vi "LC1_MS_Main_for_AEROS.vi"(0 "MS_Network_Settings":T12, 1 "Analog Output":T5(array[cluster]) {"analog info"."value" format="%#_15f"; "variation" items=["32-bit"=1, "16-bit"=2, "Single-prec"=3, "Double-prec"=4]; "mode" items=["SBO"=0, "Select"=3, "Operate"=4, "Direct"=5, "Direct No Ack"=6]}, 2 "Analog Input Index":cluster{"start":u16, "variation (Default)":T1}[](array[cluster]) {"variation (Default)" items=["Default", "32-bit with Flag", "16-bit with Flag", "32-bit without Flag", "16-bit without Flag", "Single-prec with Flag", "Double-prec with Flag"]}, 3 "Digital Input Indexes":u16[](array[numeric]), 5 "input cluster":T16={"Binary Out Mode"=6, "Binary In Variation"=0, "Analog Out Variation"=4, "Analog Out Mode"=6, "Analog In Variation"=6} {"Binary Out Mode" items=["SBO"=0, "Select"=3, "Operate"=4, "Direct"=5, "Direct No Ack"=6]; "Binary In Variation" items=["Default", "Packed Format", "With Flags"]; "Analog Out Variation" items=["32-bit"=1, "16-bit"=2, "Single-prec"=3, "Double-prec"=4]; "Analog Out Mode" items=["SBO"=0, "Select"=3, "Operate"=4, "Direct"=5, "Direct No Ack"=6]; "Analog In Variation" items=["Default", "32-bit with Flag", "16-bit with Flag", "32-bit without Flag", "16-bit without Flag", "Single-prec with Flag", "Double-prec with Flag"]}, 7 "MS_RESET":bool, 9 "MS_ENABLE":bool, 11 "Poll Enable":T13, 12 "DNP3 Session feedback":T15, 13 "Digital Output":T6[](array[typedef]) {"CROB value"."Control" items=["Nul"=0, "Pulse On"=1, "Pulse Off"=2, "Latch On"=3, "Latch Off"=4, "Close"=65, "Trip"=129]}) -> (4 "MS_SETTINGS_CHANGED":bool, 6 "MS_RESET_IND":bool, 8 "Cluster":T14, 10 "Analog Input":dbl[](array[numeric]), 14 "DNP3 Session":T15, 15 "Digital Input":bool[](array[boolean]))   [LabVIEW 2016]
uses:
  Tab_Master.ctl
  <vilib>/DNP3/DNP3_Master/Operation Mode.ctl
  <vilib>/DNP3/DNP3_Master/Poll Binary Input Variation.ctl
  <vilib>/DNP3/DNP3_Master/Analog Variation.ctl
  <vilib>/DNP3/DNP3_Master/Poll Analog Input Variation.ctl
  <vilib>/DNP3/DNP3_Master/Response Type.ctl
  <vilib>/DNP3/DNP3_Master/Start Stop.ctl
  <vilib>/DNP3/DNP3_Master/Crob With Index.ctl
  <vilib>/DNP3/DNP3_Common/crob.ctl
  <vilib>/DNP3/DNP3_Common/crob_ctrl.ctl
  <vilib>/DNP3/DNP3_Master/Analog Info.ctl
  <vilib>/Utility/error.llb/Error Cluster From Error Code.vi
  <vilib>/DNP3/DNP3_Master/Send Poll Analog Input By StartStop (Blocking).vi
  <vilib>/DNP3/DNP3_Master/Read Analog Input.vi
  <vilib>/DNP3/DNP3_Master/Send Analog Output Block (Blocking).vi
  <vilib>/DNP3/DNP3_Master/Send Poll Binary Input By StartStop (Blocking).vi
  <vilib>/DNP3/DNP3_Master/Read Binary Input.vi
  <vilib>/DNP3/DNP3_Master/Send CROB (Blocking).vi
  <vilib>/ErrorRing/Error Ring.xnode
  <vilib>/DNP3/DNP3_Master.lvlib
  <resource>/objmgr/dnp3.rc
  DNP3_Master_Station_MGCC.lvlib
  <vilib>/DNP3/DNP3_Common.lvlib
panel:
  out "PollD":T9[](array[typedef])
  out "Binary Out Mode":T4=6 items=["SBO"=0, "Select"=3, "Operate"=4, "Direct"=5, "Direct No Ack"=6]
  out "Binary In Variation":T10 items=["Default", "Packed Format", "With Flags"]
  out "Analog Out Variation":T3=4 items=["32-bit"=1, "16-bit"=2, "Single-prec"=3, "Double-prec"=4]
  out "Analog Out Mode":T4 items=["SBO"=0, "Select"=3, "Operate"=4, "Direct"=5, "Direct No Ack"=6]
  out "Analog In Variation":T1 items=["Default", "32-bit with Flag", "16-bit with Flag", "32-bit without Flag", "16-bit without Flag", "Single-prec with Flag", "Double-prec with Flag"]
  out "MS_TX_Status_Binary":T11
  out "MS_TX_Status_Analog":T11
  out "MS_RX_Status_Binary":T11
  out "MS_RX_Status_Analog":T11
  out "MS_Network_Settings_Initial":T12
  in  "En_Tx_Di":bool
  in  "En_Tx_An":bool
  in  "En_Rx_Di":bool
  in  "En_Rx_An":bool
  out "object flags":u8[](array[numeric]) format="%08b"
  in  "Channel Setting":T17
  in  "serial port":u16=1
  in  "baud rate (9600)":u32=9600
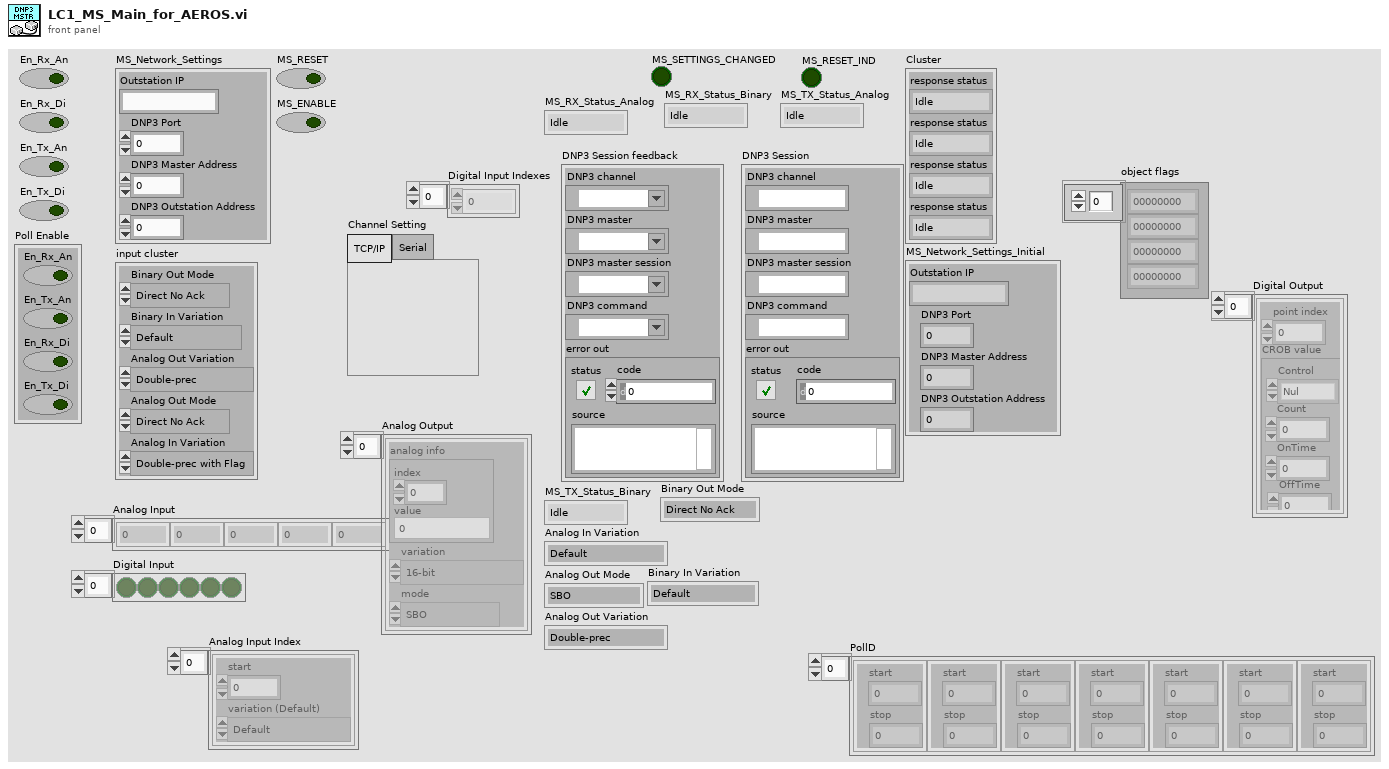
[diagram p1: front panel]
types:
  T1 = typedef "DNP3_Master.lvlib/Poll Analog Input Variation.ctl" = u8
  T2 = typedef "DNP3_Master.lvlib/Analog Info.ctl" = cluster{"index":u16, "value":dbl}
  T3 = typedef "DNP3_Master.lvlib/Analog Variation.ctl" = u8
  T4 = typedef "DNP3_Master.lvlib/Operation Mode.ctl" = u8
  T5 = cluster{"analog info":T2, "variation":T3, "mode":T4}[]
  T6 = typedef "DNP3_Master.lvlib/Crob With Index.ctl" = cluster{"point index":u16, "CROB value":T7}
  T7 = typedef "DNP3_Common.lvlib/crob.ctl" = cluster{"OnTime":u32, "Count":u8, "OffTime":u32, "Control":T8}
  T8 = typedef "DNP3_Common.lvlib/crob_ctrl.ctl" = u8
  T9 = typedef "DNP3_Master.lvlib/Start Stop.ctl" = cluster{"start":u16, "stop":u16}
  T10 = typedef "DNP3_Master.lvlib/Poll Binary Input Variation.ctl" = u8
  T11 = typedef "DNP3_Master.lvlib/Response Type.ctl" = enum16{"Idle", "Buffering", "Pending", "Success", "Failure", "Mismatch", "Status Code", "IIN", "Timeout", "Cancel"}
  T12 = cluster{"Outstation IP":string, "DNP3 Port":u16, "DNP3 Master Address":u16, "DNP3 Outstation Address":u16}
  T13 = cluster{"En_Rx_An":bool, "En_Tx_An":bool, "En_Rx_Di":bool, "En_Tx_Di":bool}
  T14 = cluster{"response status":T11, "response status":T11, "response status":T11, "response status":T11}
  T15 = cluster{"DNP3 channel":refnum<k21>, "DNP3 master":refnum<k21>, "DNP3 master session":refnum<k21>, "DNP3 command":refnum<k21>, "error out":errorcluster}
  T16 = cluster{"Binary Out Mode":T4, "Binary In Variation":T10, "Analog Out Variation":T3, "Analog Out Mode":T4, "Analog In Variation":T1}
  T17 = typedef "Tab_Master.ctl" = enum32{"TCP/IP", "Serial"}
  T18 = cluster{"Analog RX":T11, "Analog RX":T11, "Analog RX":T11, "Analog RX":T11}
  T19 = cluster{"DNP3 Master Address":u16, "DNP3 Outstation Address":u16}
  T20 = cluster{bool, "Outstation IP":string, "DNP3 Port":u16, "serial port":u16, "baud rate (9600)":u32}
  T21 = cluster{"MS_RX_Status_Analog":T11, "MS_TX_Status_Analog":T11, "MS_RX_Status_Binary":T11, "MS_TX_Status_Binary":T11}
  T22 = cluster{"DNP3 channel":refnum<k21>, "DNP3 master":refnum<k21>, "DNP3 master session":refnum<k21>, "DNP3 command":refnum<k21>, "error IO":errorcluster}
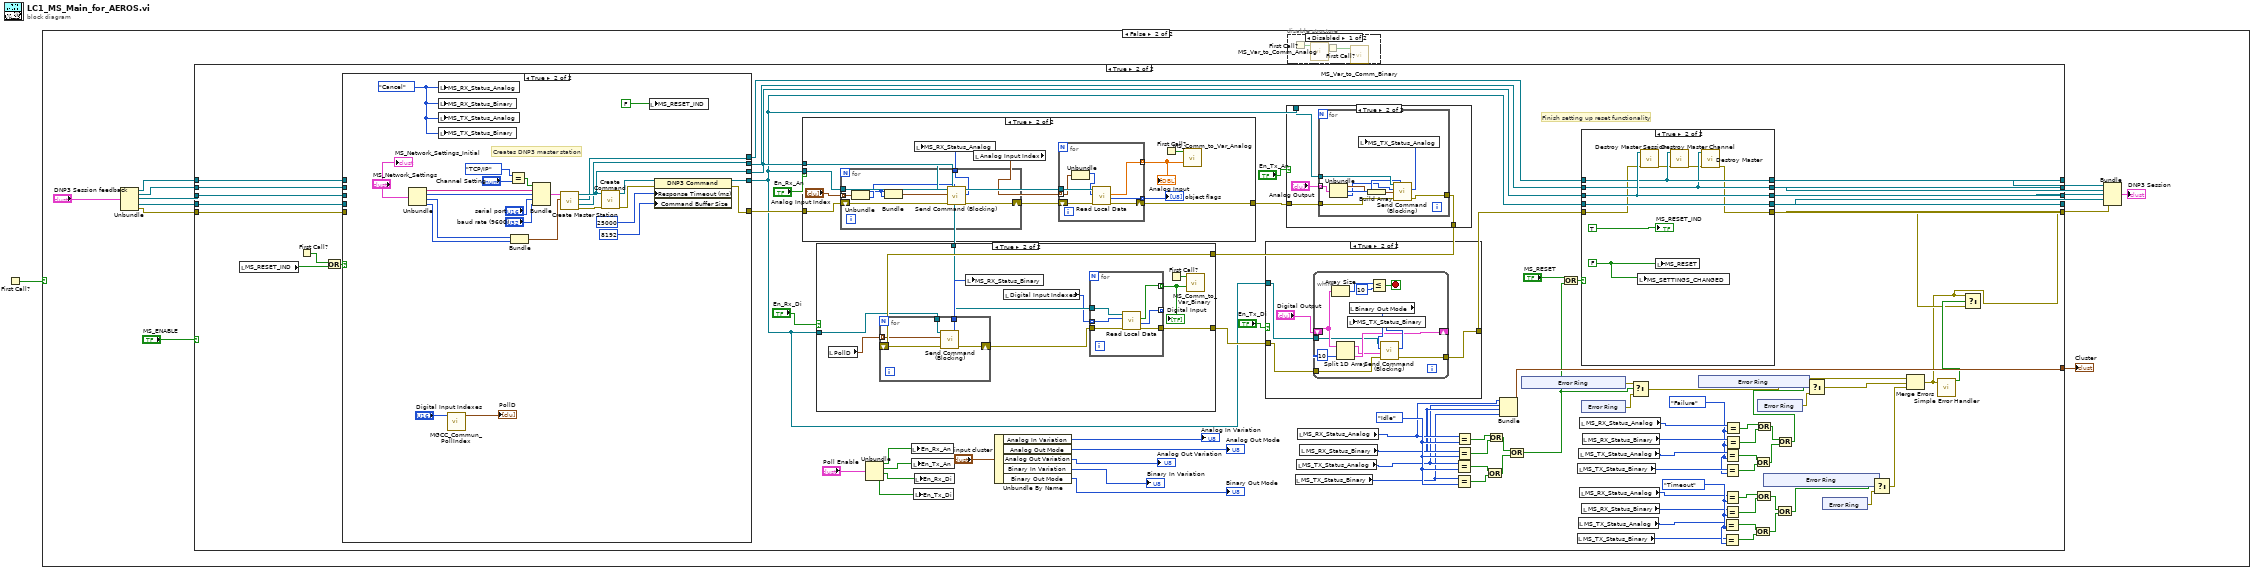
[diagram p0: block diagram]
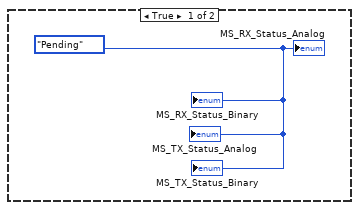
[diagram p2: hidden frame]
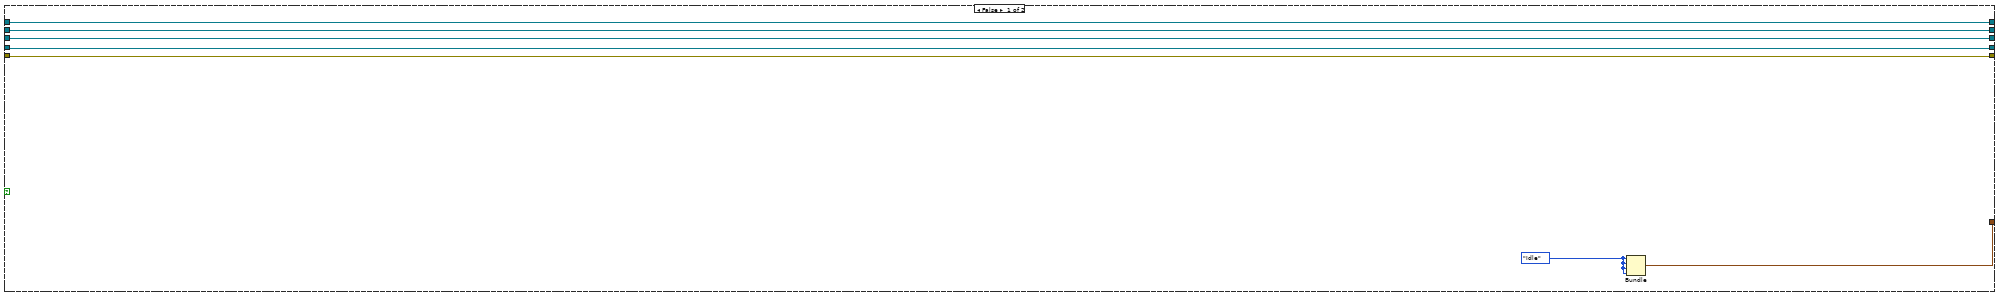
[diagram p4: hidden frame]
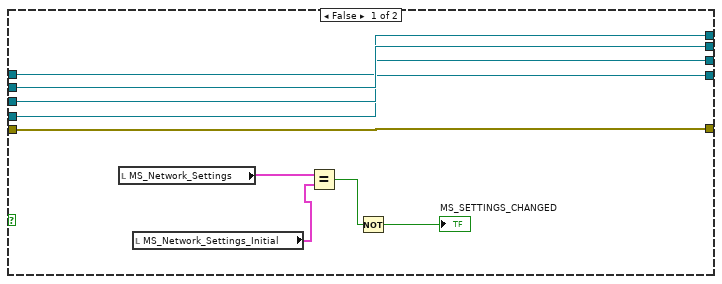
[diagram p10: hidden frame]
diagram:
  n1 = First Call?() -> (First Call?: T/F=w1:bool)
  n2 = case shown="False" w1 {
    frame True {
      w2 = Response_Type."Pending" ("LC1_MS_RX_Status_Binary")
      "MS_RX_Status_Analog" <- w2
      "MS_RX_Status_Binary" <- w2
      "MS_TX_Status_Analog" <- w2
      "MS_TX_Status_Binary" <- w2
    }
    frame False {
      n3 = Unbundle("DNP3 Session feedback") -> ("DNP3 channel"=w16:refnum<k21>, "DNP3 master"=w15:refnum<k21>, "DNP3 master session"=w13:refnum<k21>, "DNP3 command"=w14:refnum<k21>, "error out"=w12:errorcluster)
      n4 = case shown="True" "MS_ENABLE" {
        tunnel: w15 -> [w25 w109]
        tunnel: w13 -> [w24 w108]
        tunnel: w14 -> [w23 w107]
        tunnel: [w25 w105] -> w7
        tunnel: w12 -> [w22 w104]
        tunnel: [w22 w26] -> w4
        tunnel: [w24 w103] -> w6
        tunnel: [w23 w101] -> w5
        tunnel: [w21 w90] -> w8
        tunnel: w16 -> [w21 w89]
        tunnel: [w20 w85] -> w9
        frame False {
          w19 = Response_Type."Idle" ("Analog RX")
          n5 = Bundle("Analog RX"=w19, "Analog RX"=w19, "Analog RX"=w19, "Analog RX"=w19) -> (w20:T18)  [unwired: 1 in]
        }
        frame True {
          w48 = Response_Type."Timeout" ("Analog RX")
          w49 = Response_Type."Failure" ("Analog RX")
          w98 = Response_Type."Idle" ("Analog RX")
          # "Finish setting up reset functionality"
          n6 = local read "MS_RESET_IND"() -> (w71:bool)
          n7 = First Call?() -> (First Call?: T/F=w111:bool)
          n8 = Or(x=w111, y=w71) -> (x .or. y?=w110:bool)
          n9 = case shown="True" w110 {
            tunnel: [w233 w246] -> w112
            tunnel: [w231 w247] -> w81
            tunnel: [w232 w254] -> w102
            tunnel: w109 -> [w234 _]
            tunnel: w108 -> [w232 _]
            tunnel: w107 -> [w231 _]
            tunnel: [w234 w237] -> w106
            tunnel: w104 -> [w233 _]
            tunnel: [w230 w238] -> w91
            tunnel: w89 -> [w230 _]
            frame False {
              n10 = local read "MS_Network_Settings"() -> (w227:T12)
              n11 = local read "MS_Network_Settings_Initial"() -> (w226:T12)
              n12 = Equal?(x=w227, y=w226) -> (x = y?=w228:bool)
              n13 = Not(x=w228) -> (.not. x?=→"MS_SETTINGS_CHANGED":bool)
            }
            frame True {
              w239 = Response_Type."Cancel" ("LC1_MS_RX_Status_Binary")
              # "Creates DNP3 master station"
              n14 = Unbundle("MS_Network_Settings") -> ("Outstation IP"=w253:string, "DNP3 Port"=w252:u16, "DNP3 Master Address"=w251:u16, "DNP3 Outstation Address"=w250:u16)
              n15 = local write "MS_RX_Status_Analog"(w239) -> ()
              n16 = local write "MS_RX_Status_Binary"(w239) -> ()
              n17 = local write "MS_TX_Status_Analog"(w239) -> ()
              n18 = local write "MS_TX_Status_Binary"(w239) -> ()
              n19 = call "MGCC_Commun_PollIndex.vi"("Analog Input Indexes"="Digital Input Indexes") -> ("Poll"=→"PollD":T9[])  [unwired: 10 in]
              n20 = Equal?(x=Tab_Master."TCP/IP" ("Channel Setting"), y="Channel Setting") -> (x = y?=w256:bool)
              n21 = Bundle("DNP3 Master Address"=w251, "DNP3 Outstation Address"=w250) -> (w248:T19)  [unwired: 1 in]
              n22 = Bundle(w256, "Outstation IP"=w253, "DNP3 Port"=w252, "serial port"="serial port", "baud rate (9600)"="baud rate (9600)") -> (w249:T20)  [unwired: 1 in]
              n23 = call "Create Master Station.vi"("Session Cluster"=w248, "Channel Cluster"=w249) -> ("error out"=w257:errorcluster, "DNP3 master"=w237:refnum<k21>, "DNP3 channel"=w238:refnum<k21>, "DNP3 master session"=w254:refnum<k21>)  [unwired: 3 in]
              n24 = call <vilib>:"Create Command.vi"("error in (no error)"=w257, "DNP3 master session"=w254) -> ("error out"=w244:errorcluster, "DNP3 command"=w245:refnum<k21>)  [unwired: 8 in]
              n25 = local write "MS_RESET_IND"(FALSE ("MS_Comm_Reset_Ind")) -> ()
              n26 = property class="DNP3 Command"(reference=w245, error in=w244, "Response Timeout (ms)"=u32 25000 ("Misc:Response Timeout (ms)"), "Command Buffer Size"=u32 8192 ("Misc:Command Buffer Size")) -> (reference out=w247:refnum<k21>, error out=w246:errorcluster)
              "MS_Network_Settings_Initial" <- "MS_Network_Settings"
            }
          }
          n27 = case shown="True" "En_Rx_An" {
            tunnel: w112 -> [w184 w195]
            tunnel: w102 -> [_ w189]
            tunnel: w81 -> [_ w194]
            tunnel: [w184 w192] -> w84
            frame False {
            }
            frame True {
              n28 = for {
                tunnel: w194 -> [w202]
                shift-right: [w201] -> w188
                shift-left: w195 -> [w203]
                tunnel: "Analog Input Index" -> [w200] mode=indexing
                tunnel: [w196] -> w185
                n29 = Unbundle(w200) -> ("start"=w198:u16, "variation (Default)"=w199:T1)
                n30 = Bundle("start"=w198, "start"=w198) -> (w197:cluster{"start":u16, "start":u16})  [unwired: 1 in]
                n31 = call-poly <vilib>:"Send Command (Blocking).vi"("variation (Default)"=w199, "error in (no error)"=w203, "range"=w197, "DNP3 command in"=w202) -> ("error out"=w201:errorcluster, "response status"=w196:T11)  [unwired: 5 in, 1 out]
              }
              n32 = local write "MS_RX_Status_Analog"(w185) -> ()
              n33 = local read "Analog Input Index"() -> (w187:cluster{"start":u16, "variation (Default)":T1}[])
              n34 = for {
                tunnel: [w208] -> w190 mode=indexing
                tunnel: [w207] -> w193 mode=indexing
                tunnel: w189 -> [w206]
                tunnel: w187 -> [w205] mode=indexing
                shift-right: [w209] -> w192
                shift-left: w188 -> [w210]
                n35 = Unbundle(w205) -> ("start"=w204:u16)  [unwired: 1 out]
                n36 = call-poly <vilib>:"Read Local Data.vi"("error in (no error)"=w210, "point index"=w204, "DNP3 master session in"=w206) -> ("error out"=w209:errorcluster, "object flags"=w207:u8, "value"=w208:dbl)  [unwired: 5 in, 1 out]
              }
              "object flags" <- w193
              "Analog Input" <- w190
              n37 = First Call?() -> (First Call?: T/F=w191:bool)
              n38 = call "MS_Comm_to_Var_Analog.vi"("Array"=w190, "Boolean"=w191) -> ()  [unwired: 10 in]
            }
          }
          n39 = Unbundle("Poll Enable") -> ("En_Rx_An"=w76:bool, "En_Tx_An"=w75:bool, "En_Rx_Di"=w74:bool, "En_Tx_Di"=w73:bool)
          n40 = local write "En_Rx_An"(w76) -> ()
          n41 = local write "En_Tx_An"(w75) -> ()
          n42 = local write "En_Tx_Di"(w73) -> ()
          n43 = local write "En_Rx_Di"(w74) -> ()
          n44 = Unbundle By Name("input cluster") -> ("Analog In Variation"=→"Analog In Variation":T1, "Analog Out Mode"=→"Analog Out Mode":T4, "Analog Out Variation"=→"Analog Out Variation":T3, "Binary In Variation"=→"Binary In Variation":T10, "Binary Out Mode"=→"Binary Out Mode":T4)
          n45 = case shown="True" "En_Tx_An" {
            tunnel: w81 -> [_ w174]
            tunnel: w84 -> [w170 w172]
            tunnel: [w170 w173] -> w83
            frame False {
            }
            frame True {
              n46 = for {
                tunnel: [w182] -> w173
                tunnel: w174 -> [w181]
                tunnel: w172 -> [w180]
                tunnel: "Analog Output" -> [w179] mode=indexing
                n47 = Unbundle(w179) -> ("analog info"=w177:T2, "variation"=w178:T3, "mode"=w175:T4)
                n48 = Build Array(w177) -> (w176:T2[])
                n49 = call-poly <vilib>:"Send Command (Blocking).vi"("variation"=w178, "error in (no error)"=w180, "values"=w176, "mode"=w175, "DNP3 command in"=w181) -> ("error out"=w182:errorcluster, "response status"=w183:T11)  [unwired: 4 in, 1 out]
                n50 = local write "MS_TX_Status_Analog"(w183) -> ()
              }
            }
          }
          n51 = case shown="True" "En_Rx_Di" {
            tunnel: w102 -> [_ w152]
            tunnel: w81 -> [_ w150]
            tunnel: w83 -> [w148 w158]
            tunnel: [w148 w157] -> w82
            frame False {
            }
            frame True {
              n52 = local read "PollD"() -> (w149:T9[])
              n53 = for {
                tunnel: [w161] -> w153
                shift-right: [w162] -> w156
                shift-left: w158 -> [w163]
                tunnel: w150 -> [w160]
                tunnel: w149 -> [w159] mode=indexing
                n54 = call-poly <vilib>:"Send Command (Blocking).vi"("error in (no error)"=w163, "range"=w159, "DNP3 command in"=w160) -> ("error out"=w162:errorcluster, "response status"=w161:T11)  [unwired: 6 in, 1 out]
              }
              n55 = local write "MS_RX_Status_Binary"(w153) -> ()
              n56 = local read "Digital Input Indexes"() -> (w151:u16[])
              n57 = for {
                tunnel: [w169] -> w157
                tunnel: [w168] -> _ mode=indexing
                tunnel: [w167] -> w155 mode=indexing
                tunnel: w152 -> [w166]
                tunnel: w151 -> [w165] mode=indexing
                tunnel: w156 -> [w164]
                n58 = call-poly <vilib>:"Read Local Data.vi"("error in (no error)"=w164, "point index"=w165, "DNP3 master session in"=w166) -> ("error out"=w169:errorcluster, "object flags"=w168:u8, "value"=w167:bool)  [unwired: 5 in, 1 out]
              }
              "Digital Input" <- w155
              n59 = First Call?() -> (First Call?: T/F=w154:bool)
              n60 = call "MS_Comm_to_Var_Binary.vi"("Input Data"=w155, "Boolean"=w154) -> ()  [unwired: 10 in]
            }
          }
          n61 = case shown="True" "En_Tx_Di" {
            tunnel: [w131 w134] -> w100
            tunnel: w82 -> [w131 w135]
            tunnel: w81 -> [_ w132]
            frame False {
            }
            frame True {
              n62 = while {
                shift-right: [w140] -> _
                shift-left: "Digital Output" -> [w143]
                tunnel: w135 -> [w139]
                tunnel: [w138] -> w134
                tunnel: w132 -> [w136]
                stop <- w144 stop-if-true
                n63 = Array Size(array=w143) -> (size(s)=w146:i32)
                n64 = Split 1D Array(array=w143, index=10) -> (first subarray=w137:T6[], second subarray=w140:T6[])
                n65 = local read "Binary Out Mode"() -> (w142:T4)
                n66 = Less Or Equal?(x=w146, y=10) -> (x <= y?=w144:bool)
                n67 = call-poly <vilib>:"Send Command (Blocking).vi"("error in (no error)"=w139, "CROB values"=w137, "mode"=w142, "DNP3 command in"=w136) -> ("error out"=w138:errorcluster, "response status"=w141:T11)  [unwired: 5 in, 1 out]
                n68 = local write "MS_TX_Status_Binary"(w141) -> ()
              }
            }
          }
          n69 = local read "MS_TX_Status_Binary"() -> (w66:T11)
          n70 = local read "MS_TX_Status_Analog"() -> (w67:T11)
          n71 = local read "MS_RX_Status_Analog"() -> (w69:T11)
          n72 = local read "MS_RX_Status_Binary"() -> (w68:T11)
          n73 = Equal?(x=w67, y=w98) -> (x = y?=w93:bool)
          n74 = Equal?(x=w66, y=w98) -> (x = y?=w94:bool)
          n75 = Equal?(x=w69, y=w98) -> (x = y?=w95:bool)
          n76 = Equal?(x=w68, y=w98) -> (x = y?=w92:bool)
          n77 = Or(x=w93, y=w94) -> (x .or. y?=w96:bool)
          n78 = Or(x=w95, y=w92) -> (x .or. y?=w97:bool)
          n79 = Bundle("MS_RX_Status_Analog"=w69, "MS_TX_Status_Analog"=w67, "MS_RX_Status_Binary"=w68, "MS_TX_Status_Binary"=w66) -> (w85:T21)  [unwired: 1 in]
          n80 = Or(x=w97, y=w96) -> (x .or. y?=w54:bool)
          n81 = xnode "Error Ring"() -> ("error out"=w55:errorcluster)
          n82 = Or(x="MS_RESET", y=w54) -> (x .or. y?=w99:bool)
          n83 = local read "MS_TX_Status_Binary"() -> (w47:T11)
          n84 = local read "MS_TX_Status_Binary"() -> (w50:T11)
          n85 = local read "MS_TX_Status_Analog"() -> (w40:T11)
          n86 = local read "MS_TX_Status_Analog"() -> (w62:T11)
          n87 = local read "MS_RX_Status_Analog"() -> (w45:T11)
          n88 = local read "MS_RX_Status_Analog"() -> (w52:T11)
          n89 = case shown="True" w99 {
            tunnel: w106 -> [w215 w221]
            tunnel: [w215 w221] -> w105
            tunnel: w100 -> [w214 w220]
            tunnel: [w214 w217] -> w27
            tunnel: [w213 w223] -> w103
            tunnel: w102 -> [w213 w223]
            tunnel: [w212 w225] -> w101
            tunnel: w81 -> [w212 w225]
            tunnel: w91 -> [w211 w222]
            tunnel: [w211 w222] -> w90
            frame False {
            }
            frame True {
              w216 = FALSE ("MS_Comm_Reset")
              n90 = local write "MS_SETTINGS_CHANGED"(w216) -> ()
              n91 = call <vilib>:"Destroy Master Session.vi"("error in (no error)"=w220, "DNP3 master session in"=w223) -> ("error out"=w219:errorcluster)  [unwired: 8 in, 1 out]
              n92 = local write "MS_RESET"(w216) -> ()
              n93 = call <vilib>:"Destroy Master Channel.vi"("error in (no error)"=w219, "DNP3 channel in"=w222) -> ("error out"=w218:errorcluster)  [unwired: 8 in, 1 out]
              n94 = call <vilib>:"Destroy Master.vi"("error in (no error)"=w218, "DNP3 master"=w221) -> ("error out"=w217:errorcluster)  [unwired: 9 in]
              "MS_RESET_IND" <- TRUE ("MS_Comm_Reset_Succesful")
            }
          }
          n95 = xnode "Error Ring"() -> ("error out"=w56:errorcluster)
          n96 = local read "MS_RX_Status_Binary"() -> (w46:T11)
          n97 = local read "MS_RX_Status_Binary"() -> (w51:T11)
          n98 = Select(t=w55, s=w54, f=w56) -> (s? t:f=w31:errorcluster)
          n99 = xnode "Error Ring"() -> ("error out"=w37:errorcluster)
          n100 = Equal?(x=w40, y=w48) -> (x = y?=w42:bool)
          n101 = Equal?(x=w47, y=w48) -> (x = y?=w43:bool)
          n102 = Equal?(x=w62, y=w49) -> (x = y?=w60:bool)
          n103 = Equal?(x=w50, y=w49) -> (x = y?=w59:bool)
          n104 = Equal?(x=w45, y=w48) -> (x = y?=w44:bool)
          n105 = Equal?(x=w46, y=w48) -> (x = y?=w41:bool)
          n106 = Equal?(x=w52, y=w49) -> (x = y?=w53:bool)
          n107 = Equal?(x=w51, y=w49) -> (x = y?=w61:bool)
          n108 = Or(x=w42, y=w43) -> (x .or. y?=w38:bool)
          n109 = Or(x=w60, y=w59) -> (x .or. y?=w58:bool)
          n110 = Or(x=w44, y=w41) -> (x .or. y?=w39:bool)
          n111 = Or(x=w53, y=w61) -> (x .or. y?=w57:bool)
          n112 = xnode "Error Ring"() -> ("error out"=w36:errorcluster)
          n113 = xnode "Error Ring"() -> ("error out"=w34:errorcluster)
          n114 = Or(x=w39, y=w38) -> (x .or. y?=w32:bool)
          n115 = Or(x=w57, y=w58) -> (x .or. y?=w33:bool)
          n116 = Select(t=w37, s=w33, f=w36) -> (s? t:f=w30:errorcluster)
          n117 = xnode "Error Ring"() -> ("error out"=w35:errorcluster)
          n118 = Select(t=w34, s=w32, f=w35) -> (s? t:f=w29:errorcluster)
          n119 = Merge Errors(w31, w30, w29) -> (w26:errorcluster)
          n120 = call <vilib>:"Simple Error Handler.vi"("error in (no error)"=w26) -> ("error?"=w28:bool)  [unwired: 4 in, 4 out]
          n121 = Select(t=w26, s=w28, f=w27) -> ()  [unwired: 1 out]
        }
      }
      "Cluster" <- w9
      n122 = disable-structure shown="Disabled" {
        frame Disabled {
          n123 = First Call?() -> (First Call?: T/F=w18:bool)
          n124 = call "MS_Var_to_Comm_Analog.vi"("Boolean"=w18) -> ()  [unwired: 11 in]
          n125 = First Call?() -> (First Call?: T/F=w17:bool)
          n126 = call "MS_Var_to_Comm_Binary.vi"("Boolean"=w17) -> ()  [unwired: 10 in, 1 out]
        }
        frame Enabled {
        }
      }
      n127 = Bundle("DNP3 channel"=w8, "DNP3 master"=w7, "DNP3 master session"=w6, "DNP3 command"=w5, "error IO"=w4) -> (→"DNP3 Session":T22)  [unwired: 1 in]
    }
  }
